vi "RichToFlatni_measurementlink_discovery_v1_ResolveServiceRequest.vi"(5 "OutputClusterType":T1, 11 "InputCluster":T2) -> (3 "OutputCluster":T1)   [LabVIEW 2021, in "Measurement Plugin Discovery Client.lvlib"]
uses:
  Measurement Plugin Discovery Client.lvlib
  ni_measurementlink_discovery_v1_ResolveServiceRequest.ctl
  ni_measurementlink_discovery_v1_ResolveServiceRequest_Flat.ctl
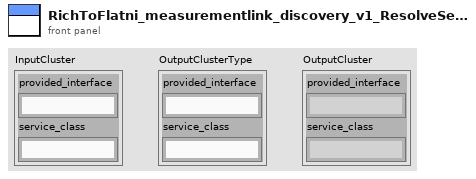
[diagram p1: front panel]
types:
  T1 = typedef "Measurement Plugin Discovery Client.lvlib/ni_measurementlink_discovery_v1_ResolveServiceRequest_Flat.ctl" = cluster{"provided_interface":string, "service_class":string}
  T2 = typedef "Measurement Plugin Discovery Client.lvlib/ni_measurementlink_discovery_v1_ResolveServiceRequest.ctl" = cluster{"provided_interface":string, "service_class":string}
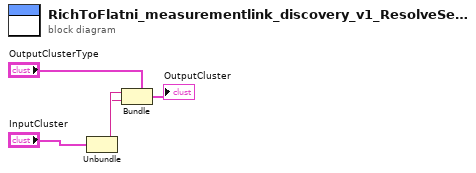
[diagram p0: block diagram]
diagram:
  n1 = Unbundle "Unbundle"("InputCluster") -> ("provided_interface"=w2:string, "service_class"=w1:string)
  n2 = Bundle "Bundle"(cluster="OutputClusterType", "provided_interface"=w2, "service_class"=w1) -> (→"OutputCluster":T1)
